vi "Sequence Throw away.vi"(8 "error in (no error)":errorcluster, 9 "Intruction Cluster":T1 {"Control" items=["Setpoint", "Pump %"]}, 10 "Found?":bool, 11 "Queue in":refnum<queue>) -> (0 "error out":errorcluster, 3 "Module":string)   [LabVIEW 2021, in "Sequencing Library.lvlib"]
uses:
  Sequencing Library.lvlib
  Squence Update Cluster.ctl
  support/Message Queue/Enqueue Message (Single).vi
  support/Message Queue/Message Cluster.ctl
  Squence Control.ctl
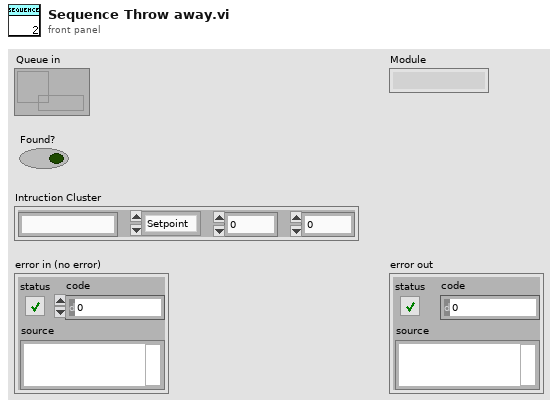
[diagram p1: front panel]
types:
  T1 = typedef "Sequencing Library.lvlib/Squence Control.ctl" = cluster{"Module":string, "Control":u16, "Value":dbl, "Wait (sec)":dbl}
  T2 = typedef "Sequencing Library.lvlib/Squence Update Cluster.ctl" = cluster{"Auto?":bool, "Manual Entry":dbl, "Setpoint":dbl}
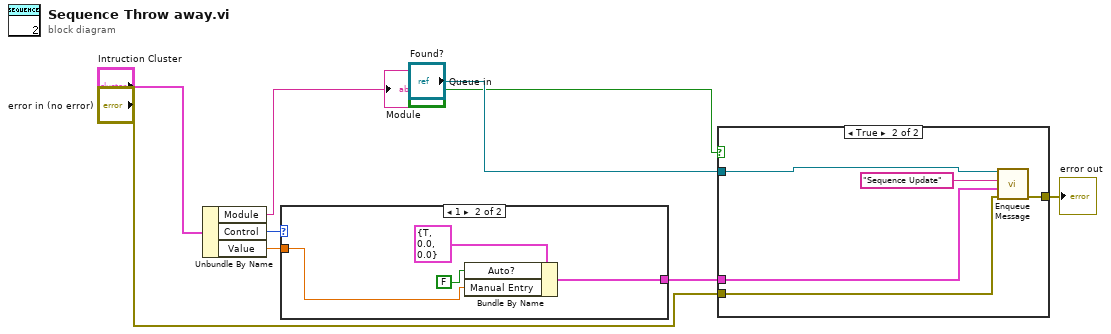
[diagram p0: block diagram]
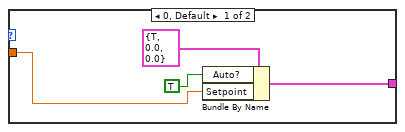
[diagram p3: hidden frame]
diagram:
  n1 = Unbundle By Name("Intruction Cluster") -> ("Module"=→"Module":string, "Control"=w1:u16, "Value"=w2:dbl)
  n2 = case shown="1" w1 {
    tunnel: [w11 w15] -> w7
    tunnel: w2 -> [w10 w14]
    frame 0, Default {
      n3 = Bundle By Name(cluster=T2 {"Auto?"=TRUE, "Manual Entry"=0.0, "Setpoint"=0.0}, "Auto?"=TRUE, "Setpoint"=w10) -> (w11:T2)
    }
    frame 1 {
      n4 = Bundle By Name(cluster=T2 {"Auto?"=TRUE, "Manual Entry"=0.0, "Setpoint"=0.0}, "Auto?"=FALSE, "Manual Entry"=w14) -> (w15:T2)
    }
  }
  n5 = case shown="True" "Found?" {
    tunnel: "error in (no error)" -> [w18 w23]
    tunnel: w7 -> [_ w22]
    tunnel: [w18 w20] -> w8
    tunnel: "Queue in" -> [_ w19]
    frame False {
    }
    frame True {
      n6 = call-poly "Enqueue Message.vi"("error in (no error)"=w23, "Message Data"=w22, "Message"="Sequence Update", "Message Queue"=w19) -> ("error out"=w20:errorcluster)  [unwired: 6 in, 1 out]
    }
  }
  "error out" <- w8
